vi "SMT_Material Modify.vi"(0 "Traceability 引用句柄":refnum<k24>, 1 "Barcode":string, 2 "RepMaterialNo":string, 5 "LoadID":string, 7 "ItemID":string, 9 "CellID":string, 11 "error in (no error)":errorcluster caption="错误输入（无错误）", 12 "MaterialNo":string, 13 "OperatorName":string) -> (4 "Traceability 引用句柄输出":refnum<k24>, 6 "SMT_MaterialModify":string, 15 "error out":errorcluster caption="错误输出")   [LabVIEW 2014, in "Traceability.lvlib"]
uses:
  D:/webservice/Traceability.dll
  Traceability.dll
  Traceability.lvlib
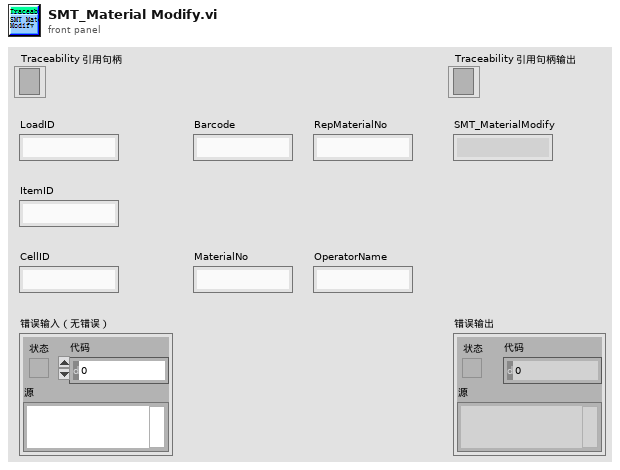
[diagram p1: front panel]
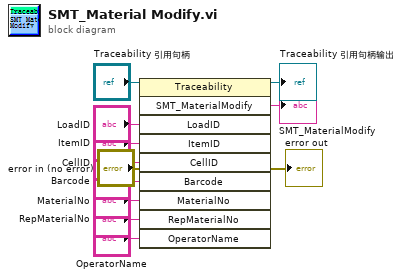
[diagram p0: block diagram]
diagram:
  n1 = invoke class="Traceability" method="SMT_MaterialModify"(reference="Traceability 引用句柄", error in="error in (no error)", "LoadID"="LoadID", "ItemID"="ItemID", "CellID"="CellID", "Barcode"="Barcode", "MaterialNo"="MaterialNo", "RepMaterialNo"="RepMaterialNo", "OperatorName"="OperatorName") -> (reference out=→"Traceability 引用句柄输出":refnum<k24>, error out=→"error out":errorcluster, "SMT_MaterialModify"=→"SMT_MaterialModify":string)  [unwired: 1 in, 7 out]
